vi "LFCSimShutter.vi"(8 "error in (no error)":errorcluster, 11 "LFCSim":T1) -> (0 "error out":errorcluster, 3 "LFCSim out":T1)   [LabVIEW 2016]
uses:
  Controls/Shutter Data.ctl
  Controls/Shutter States.ctl
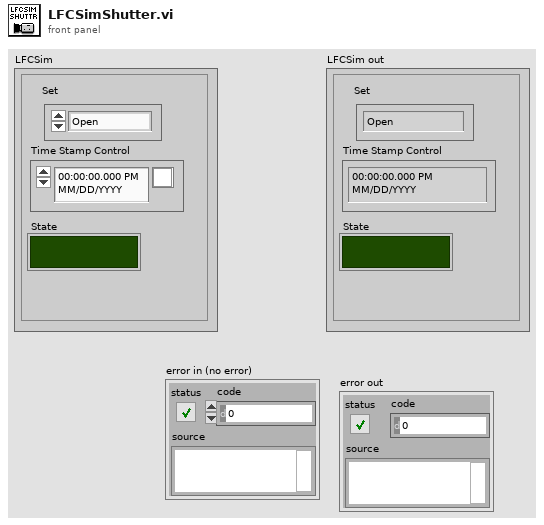
[diagram p1: front panel]
types:
  T1 = typedef "Shutter Data.ctl" = cluster{"Time Stamp Control":timestamp, "State":bool, "Set":T2}
  T2 = typedef "Shutter States.ctl" = enum16{"Open", "Close", "Wait", "Off", "Arm", "Idle"}
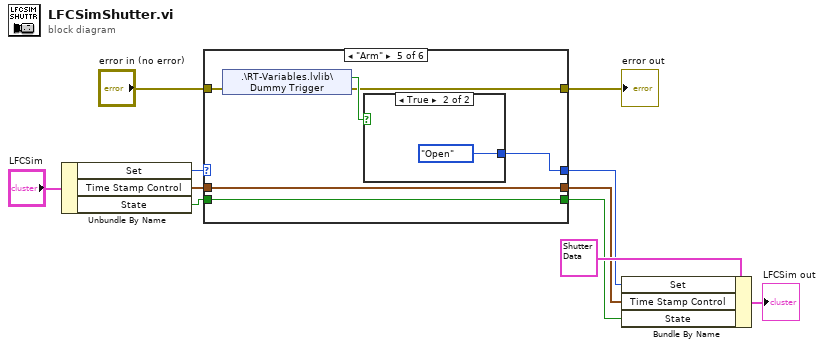
[diagram p0: block diagram]
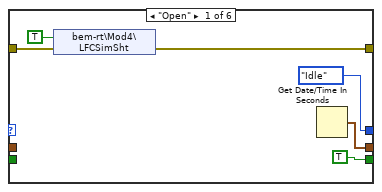
[diagram p2: hidden frame]
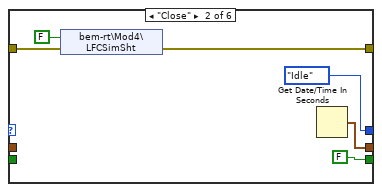
[diagram p3: hidden frame]
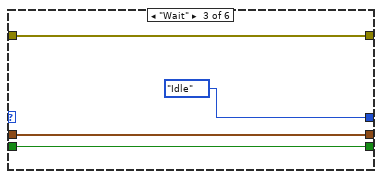
[diagram p4: hidden frame]
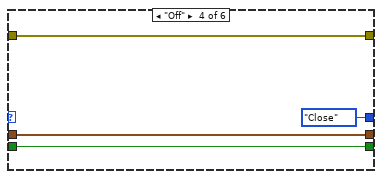
[diagram p5: hidden frame]
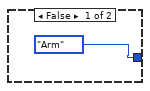
[diagram p6: hidden frame]
diagram:
  n1 = Unbundle By Name("LFCSim") -> ("Set"=w11:T2, "Time Stamp Control"=w8:timestamp, "State"=w6:bool)
  n2 = case shown="\"Arm\"" w11 {
    selector: w11 -> [_ _ _ _ _ w43]
    tunnel: [Shutter_States."Idle" ("Set") Shutter_States."Idle" ("Set") Shutter_States."Idle" ("Set") Shutter_States."Close" ("Set") w36 w43] -> w2
    tunnel: w8 -> [_ _ w24 w30 w32 w42]
    tunnel: [w17 w23 w24 w30 w32 w42] -> w7
    tunnel: w6 -> [_ _ w25 w29 w35 w41]
    tunnel: [TRUE ("State") FALSE ("State") w25 w29 w35 w41] -> w1
    tunnel: [w14 w19 w27 w28 w34 w40] -> w5
    tunnel: "error in (no error)" -> [w15 w20 w27 w28 w33 w40]
    frame "Open" {
      n3 = shared-variable "bem-rt\\Mod4\\LFCSimSht"(TRUE ("SciShtPwr"), error in=w15) -> (error out=w14:errorcluster)
      n4 = Get Date/Time In Seconds() -> (seconds since 1Jan1904=w17:timestamp)
    }
    frame "Close" {
      n5 = shared-variable "bem-rt\\Mod4\\LFCSimSht"(FALSE ("SciShtPwr"), error in=w20) -> (error out=w19:errorcluster)
      n6 = Get Date/Time In Seconds() -> (seconds since 1Jan1904=w23:timestamp)
    }
    frame "Wait" {
    }
    frame "Off" {
    }
    frame "Arm" {
      n7 = shared-variable ".\\RT-Variables.lvlib\\Dummy Trigger"(error in=w33) -> (w37:bool, error out=w34:errorcluster)
      n8 = case shown="True" w37 {
        tunnel: [Shutter_States."Arm" ("Set") Shutter_States."Open" ("Set")] -> w36
        frame False {
        }
        frame True {
        }
      }
    }
    frame "Idle" {
    }
  }
  "error out" <- w5
  n9 = Bundle By Name(cluster=T1 {"Time Stamp Control"=timestamp(0 s since 1904-01-01), "State"=FALSE, "Set"=enum."Open"} ("Shutter"), "Set"=w2, "Time Stamp Control"=w7, "State"=w1) -> (→"LFCSim out":T1)
